vi "CreateTDMSFileExample.vi"() -> ()   [LabVIEW 2017]
uses:
  <vilib>/addons/InsightCM/Utilities/Tdms/Tdms.lvlib
  <vilib>/addons/InsightCM/Utilities/GlobalConfiguration/GlobalConfiguration.lvlib
  <vilib>/measure/NI_MABase.lvlib
panel:
  out "Created TDMS File":path
  # "Run this VI and inspect the file below"
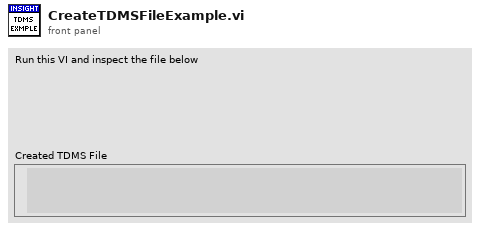
[diagram p1: front panel]
types:
  T1 = enum16{"open", "open or create", "create or replace", "create", "open (read-only)"}
  T2 = typedef "R2_DeviceModel.ctl" = cluster{"Device":T3, "Channels":T11[], "Tags":T13[]}
  T3 = typedef "R2_Device.ctl" = cluster{"Id":string, "Name":string, "DeviceType":string, "HardwareName":string, "IpAddress":string, "HardwareInfo":T4[], "ApplicationType":string, "ApplicationVersion":string, "EquipmentIds":string[], "ConfigurationVersion":string, "State":T5, "Properties":T4[], "DataGroups":T6[], "BurstModeTrigger":T10}
  T4 = typedef "KeyValuePair.ctl" = cluster{"Key":string, "Value":string}
  T5 = typedef "DeviceState.ctl" = cluster{"Disabled":bool}
  T6 = typedef "R2_DataGroup.ctl" = cluster{"Name":string, "OperatingStates":T7[], "Properties":T4[], "EquipmentIds":string[], "AssetNodeId":string}
  T7 = typedef "OperatingState.ctl" = cluster{"Name":string, "Properties":T4[], "Triggers":T8[]}
  T8 = typedef "Trigger.ctl" = cluster{"Type":string, "Expression":string, "Conditions":T9[]}
  T9 = typedef "Condition.ctl" = cluster{"Source":string, "Type":string, "Operator":string, "CompareTo":string, "DwellSeconds":dbl}
  T10 = typedef "BurstModeTrigger.ctl" = cluster{"Trigger":T8, "SampleRate":string, "AcquisitionLength":string}
  T11 = typedef "R2_Channel.ctl" = cluster{"Id":string, "DeviceId":string, "Name":string, "ChannelType":string, "HardwareKey":string, "HardwareChannel":string, "DataGroup":string, "Keywords":string[], "EquipmentIds":string[], "Properties":T4[], "Metrics":T12[], "AssetNodeId":string, "MeasType":string, "AssetName":string}
  T12 = typedef "Metric.ctl" = cluster{"Id":string, "Name":string, "Unit":string, "Properties":T4[], "MetricDefinitionInstanceId":string}
  T13 = typedef "Tag.ctl" = cluster{"Id":string, "Path":string, "Name":string, "Datatype":string, "Props":T4[], "Keywords":string[]}
  T14 = typedef "Equipment.ctl" = cluster{"Id":string, "ParentId":string, "Levelname":string, "Name":string, "Properties":T4[]}
  T15 = typedef "Tdms.lvlib/Property.ctl" = cluster{"Name":string, "Value":variant}
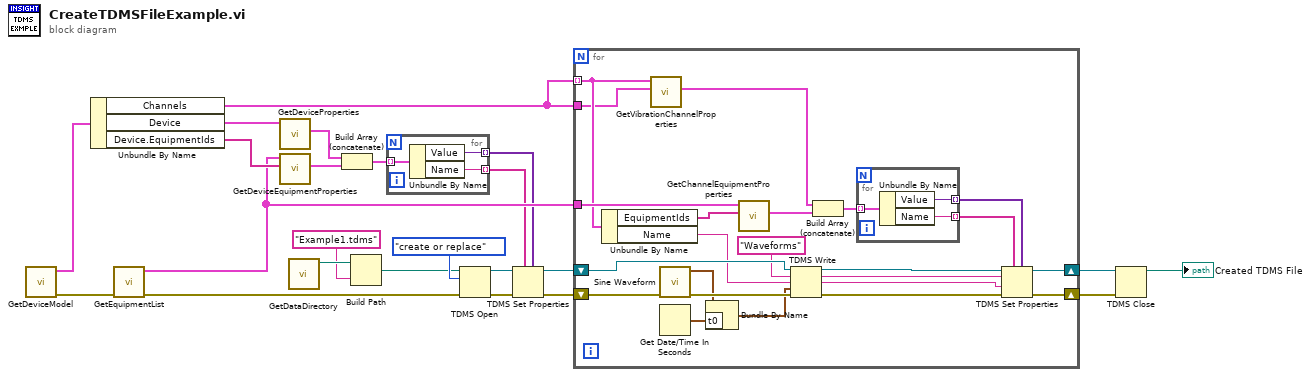
[diagram p0: block diagram]
diagram:
  n1 = call <vilib>:"GetDeviceModel.vi"() -> ("error out"=w19:errorcluster, "device model"=w20:T2)  [unwired: 9 in, 1 out]
  n2 = Unbundle By Name(w20) -> ("Channels"=w21:T11[], "Device"=w23:T3, "Device.EquipmentIds"=w22:string[])
  n3 = call <vilib>:"GetEquipmentList.vi"("error in (no error)"=w19) -> ("error out"=w18:errorcluster, "equipment list"=w17:T14[])  [unwired: 8 in, 1 out]
  n4 = call <vilib>:"GetDeviceProperties.vi"("device"=w23) -> ("tdms properties"=w13:T15[])  [unwired: 10 in]
  n5 = call <vilib>:"GetDeviceEquipmentProperties.vi"("equipment Ids"=w22, "equipment list"=w17) -> ("tdms properties"=w12:T15[])  [unwired: 9 in]
  n6 = call <vilib>:"GetDataDirectory.vi"() -> ("data directory"=w4:path)  [unwired: 10 in, 1 out]
  n7 = Build Array (concatenate)(w13, w12) -> (w11:T15[])
  n8 = Build Path(base path=w4, name or relative path="Example1.tdms" ("format string")) -> (appended path=w3:path)
  n9 = for {
    tunnel: w11 -> [w26] mode=indexing
    tunnel: [w25] -> w10 mode=indexing
    tunnel: [w24] -> w9 mode=indexing
    n10 = Unbundle By Name(w26) -> ("Value"=w24:variant, "Name"=w25:string)
  }
  n11 = TDMS Open(8:w18, 10:T1."create or replace" ("operation (0:open)"), 11:w3) -> (0:w14:errorcluster, 3:w15:refnum<k34>)  [unwired: 4 in]
  n12 = TDMS Set Properties(5:w9, 7:w10, 8:w14, 11:w15) -> (0:w8:errorcluster, 3:w7:refnum<k34>)  [unwired: 2 in, 2 out]
  n13 = for {
    shift-right: [w43] -> w5
    shift-left: w8 -> [w38]
    tunnel: w21 -> [w31]
    tunnel: w17 -> [w48]
    shift-right: [w42] -> w6
    shift-left: w7 -> [w40]
    tunnel: w21 -> [w32] mode=indexing
    n14 = Unbundle By Name(w32) -> ("EquipmentIds"=w49:string[], "Name"=w36:string)
    n15 = call <vilib>:"GetVibrationChannelProperties.vi"("all channels"=w31, "channel"=w32) -> ("TDMS properties"=w30:T15[])  [unwired: 9 in]
    n16 = call <vilib>:"Sine Waveform.vi"("error in (no error)"=w38) -> ("error out"=w37:errorcluster, "signal out"=w29:waveform(dbl))  [unwired: 9 in]
    n17 = Get Date/Time In Seconds() -> (seconds since 1Jan1904=w27:timestamp)
    n18 = Bundle By Name(cluster=w29, "t0"=w27) -> (w28:waveform(dbl))
    n19 = call <vilib>:"GetChannelEquipmentProperties.vi"("equipment Ids"=w49, "equipment list"=w48) -> ("TDMS properties"=w47:T15[])  [unwired: 9 in]
    n20 = TDMS Write(0:w40, 5:"Waveforms" ("group name in (Untitled)"), 7:w36, 9:w28, 11:w37) -> (4:w39:refnum<k34>, 6:w34:string, 8:w33:string, 15:w41:errorcluster)  [unwired: 1 in]
    n21 = Build Array (concatenate)(w30, w47) -> (w46:T15[])
    n22 = for {
      tunnel: w46 -> [w52] mode=indexing
      tunnel: [w51] -> w45 mode=indexing
      tunnel: [w50] -> w44 mode=indexing
      n23 = Unbundle By Name(w52) -> ("Value"=w50:variant, "Name"=w51:string)
    }
    n24 = TDMS Set Properties(5:w44, 7:w45, 8:w41, 9:w33, 10:w34, 11:w39) -> (0:w43:errorcluster, 3:w42:refnum<k34>)  [unwired: 2 out]
  }
  n25 = TDMS Close(8:w5, 11:w6) -> (3:→"Created TDMS File":path)  [unwired: 1 out]
